vi "test Actor Core Lookup.vi"(8 "error in (no error)":errorcluster, 11 "TestCase in":refnum<class "Monitor Test.lvclass">) -> (0 "error out":errorcluster, 3 "TestCase out":refnum<class "Monitor Test.lvclass">)   [LabVIEW 2017, in "Monitor Test.lvclass"]
uses:
  Monitor Test.lvclass
  Source/Monitor Data/Actor Data.ctl
  <vilib>/ActorFramework/Message Enqueuer/Message Enqueuer.lvclass
  Test Actor/Test Actor.lvclass
  C:/Program Files (x86)/National Instruments/LabVIEW 2017/vi.lib/ActorFramework/Actor/Actor.lvclass
  <vilib>/ActorFramework/Message Enqueuer/Message Enqueuer.lvclass/Message Enqueuer.ctl
  <vilib>/ActorFramework/Message Enqueuer/Enqueue.vi
  <vilib>/ActorFramework/Stop Msg/Stop Msg.lvclass
  C:/Program Files (x86)/National Instruments/LabVIEW 2017/vi.lib/ActorFramework/Message/Message.lvclass
  <vilib>/ActorFramework/Message Priority Queue/Priority Enqueue.vi
  <vilib>/ActorFramework/Actor/Actor.lvclass
  Debug Monitor/Debug Monitor.lvclass
  Source/Monitor Data/Monitor Data.lvclass
panel:
  out "Actor Data":T1={"Actor Type"="", "Actor Cores"=[], "Self"=refnum, "Caller"=refnum, "Actor Label"="", "Last Ping"=-1.0}
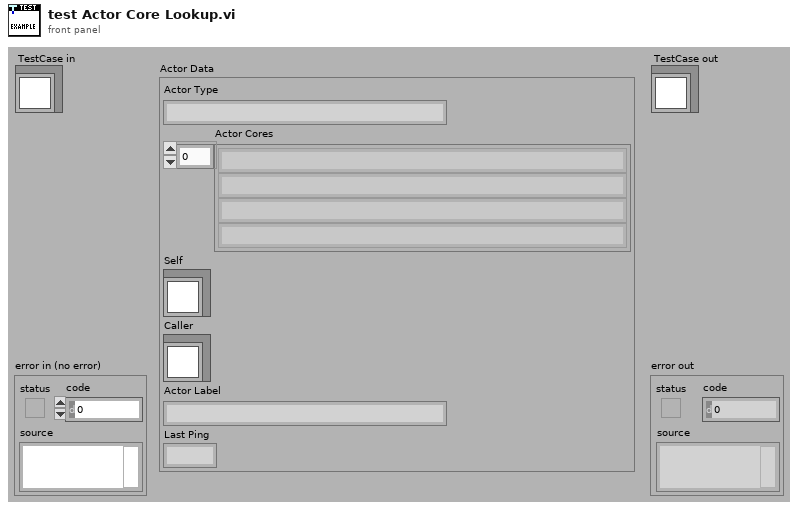
[diagram p1: front panel]
types:
  T1 = typedef "MGI-Monitored Actor Core.lvlib/Monitor Data.lvclass/Actor Data.ctl" = cluster{"Actor Type":string, "Actor Cores":string[], "Self":refnum<class "Message Enqueuer.lvclass">, "Caller":refnum<class "Message Enqueuer.lvclass">, "Actor Label":string, "Last Ping":dbl}
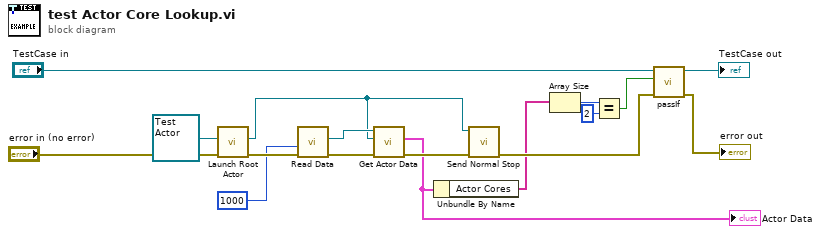
[diagram p0: block diagram]
diagram:
  n1 = call <vilib>:"Launch Root Actor.vi"("error in (no error)"="error in (no error)", "Actor"=refnum<class "Test Actor.lvclass"> refnum ("Test Actor.lvclass")) -> ("error out"=w17:errorcluster, "Actor's Enqueuer"=w12:refnum<class "Message Enqueuer.lvclass">)  [unwired: 8 in]
  n2 = call "Read Data.vi"("error in (no error)"=w17, "timeout in ms (-1)"=1000) -> ("error out"=w13:errorcluster, "Monitor Data"=w14:refnum<class "Monitor Data.lvclass">)  [unwired: 7 in, 1 out]
  n3 = call "Get Actor Data.vi"("error in (no error)"=w13, "Actor's Self Q"=w12, "Monitor Data in"=w14) -> ("error out"=w11:errorcluster, "Actor Data"=w2:T1)  [unwired: 5 in, 2 out]
  "Actor Data" <- w2
  n4 = Unbundle By Name(w2) -> ("Actor Cores"=w1:string[])
  n5 = call <vilib>:"Send Normal Stop.vi"("error in (no error)"=w11, "Message Enqueuer"=w12) -> ("error out"=w16:errorcluster)  [unwired: 9 in]
  n6 = Array Size(array=w1) -> (size(s)=w5:i32)
  n7 = Equal?(x=w5, y=2) -> (x = y?=w3:bool)
  n8 = call-dynamic "passIf.vi"("error in (no error)"=w16, "pass"=w3, "TestCase in"="TestCase in") -> ("error out"=→"error out":errorcluster, "TestCase out"=→"TestCase out":refnum<class "Monitor Test.lvclass">)  [unwired: 7 in]
